vi "TestVI.vi"() -> ()   [LabVIEW 2017]
panel:
  out "appended path":path
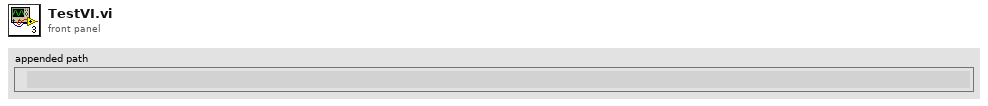
[diagram p1: front panel]
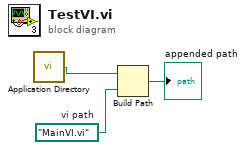
[diagram p0: block diagram]
diagram:
  w2 = path "MainVI.vi"  # vi path
  n1 = call <vilib>:"Application Directory.vi"() -> ("Application Directory"=w3:path)
  n2 = Build Path(base path=w3, name or relative path=w2) -> (appended path=→"appended path":path)
